vi "PH_AxisGUI_BaseClass.Find Axes of Controllers.vi"(0 "Own Motion Instance (N/A)":string="N/A", 1 "GUI Instance (N/A)":string="N/A", 2 "PH_AxisGUI_6P":bool=TRUE, 3 "PH_Sixpack_Switch":bool=TRUE, 4 "PH_Waveplate-GUI_6P":bool=TRUE, 5 "error in":errorcluster, 7 "PH_4_Pos_Selector":bool=TRUE, 9 "PH_Revolver-GUI_6P":bool=TRUE) -> (17 "Result":T2(array[cluster]), 19 "error out":errorcluster)   [LabVIEW 2014, in "PH_AxisGUI_BaseClass.lvlib"]
doc: "This VI reads out the database: It searches for all Motion and related GUI instances. \n\nIf \"GUI Instance (N/A)\" is connected, THIS GUI instance is kicked out of the Results.\n\nIf \"Own 6P Controller Instance (N/A)\" is connected, only GUIs of this THIS instances are given out; otherwise all.\n\nThe results are a multi-line three column olutput: \n1. columns is the motion instance,\n2. column is the axis GUI name, \n3. column is the motor number."
uses:
  PH_AxisGUI_BaseClass.lvlib
  PH_Stepmotor_BaseClass/PH_Stepmotor_BaseClass.Axis Address.ctl
  PH_Common/PH_Common.lvlib
  PH_Stepmotor_BaseClass/PH_Stepmotor_BaseClass.lvlib
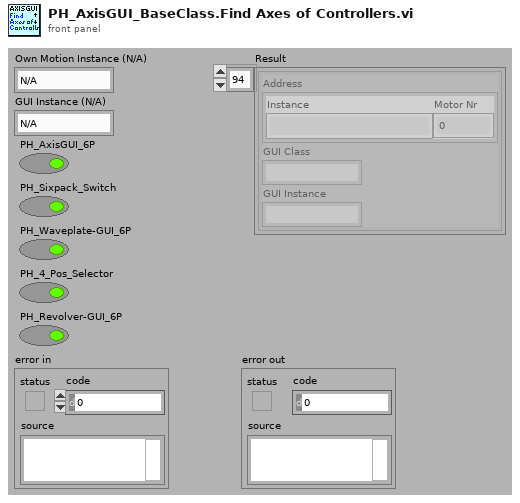
[diagram p1: front panel]
types:
  T1 = typedef "PH_Stepmotor_BaseClass.lvlib/PH_Stepmotor_BaseClass.Axis Address.ctl" = cluster{"Instance":string, "Motor Nr":i32}
  T2 = cluster{"Address":T1, "GUI Class":string, "GUI Instance":string}[]
  T3 = cluster{"Address":T1, "GUI Class":string, "GUI Instance":string}
  T4 = typedef "PH_AxisGUI_BaseClass.lvlib/PH_AxisGUI_BaseClass.Database Entry.ctl" = cluster{"Address":T1, "Name":string, "Label \"Back\"":string, "Labell \"Forth\"":string}
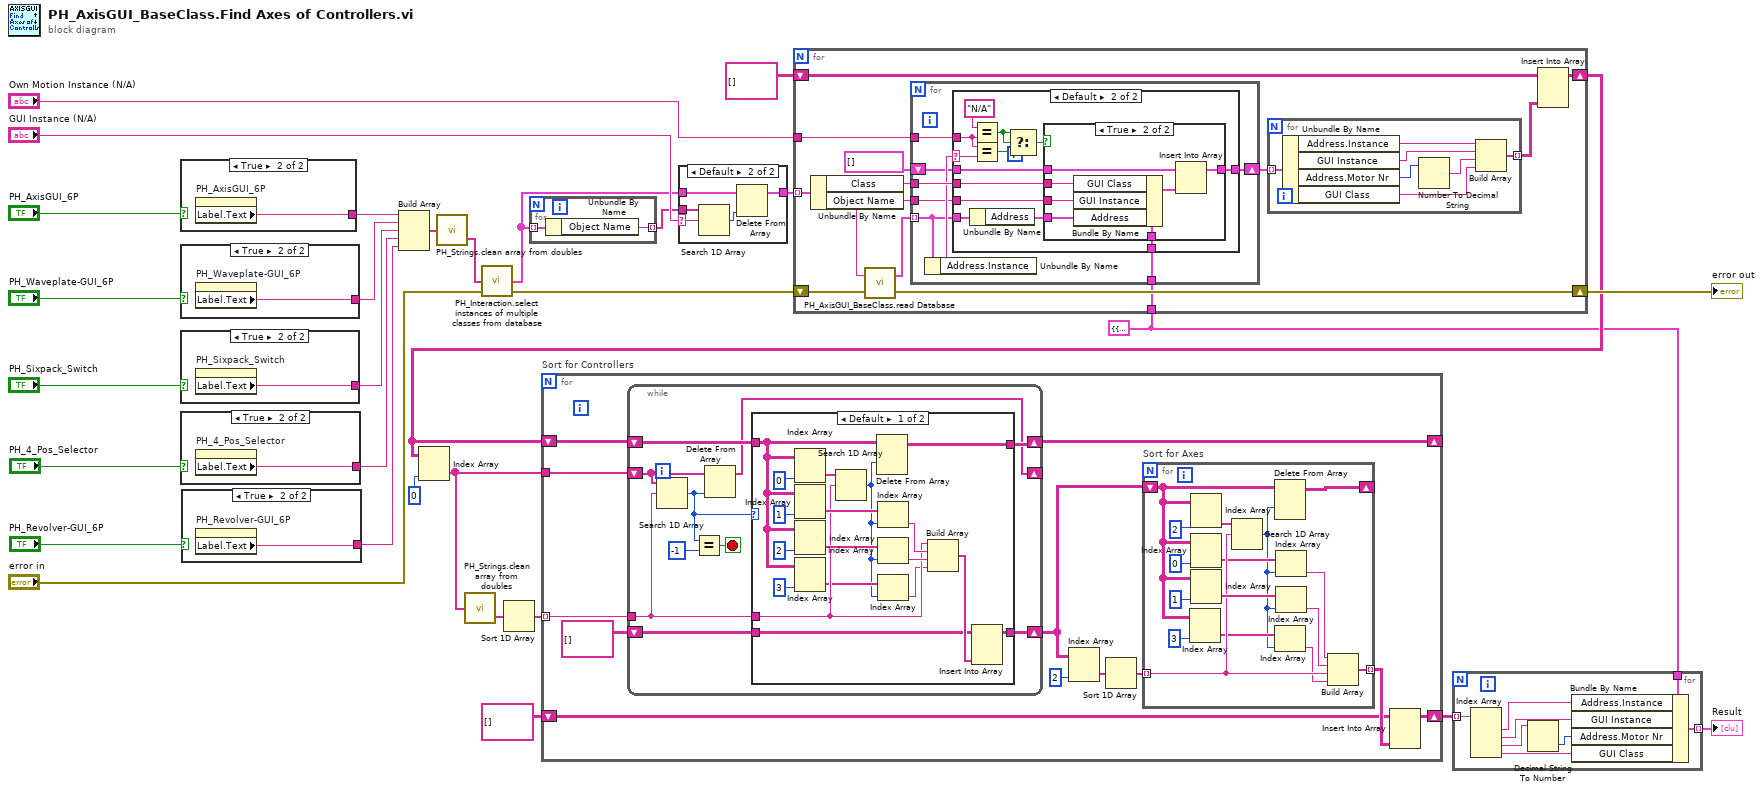
[diagram p0: block diagram]
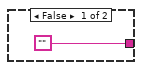
[diagram p3: hidden frame]
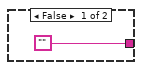
[diagram p4: hidden frame]
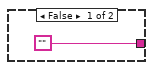
[diagram p5: hidden frame]
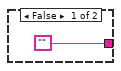
[diagram p6: hidden frame]
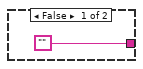
[diagram p7: hidden frame]
diagram:
  w3 = T3 {"Address"={"Instance"="N/A", "Motor Nr"=0}, "GUI Class"="", "GUI Instance"=""}
  n1 = case shown="True" "PH_AxisGUI_6P" {
    tunnel: ["" w32] -> w16
    frame False {
    }
    frame True {
      n2 = property on="PH_AxisGUI_6P" class="Bool (strict)"() -> ("Label.Text"=w32:string)  [unwired: 2 in, 2 out]
    }
  }
  n3 = case shown="True" "PH_Waveplate-GUI_6P" {
    tunnel: ["" w34] -> w20
    frame False {
    }
    frame True {
      n4 = property on="PH_Waveplate-GUI_6P" class="Bool (strict)"() -> ("Label.Text"=w34:string)  [unwired: 2 in, 2 out]
    }
  }
  n5 = case shown="True" "PH_Sixpack_Switch" {
    tunnel: ["" w36] -> w17
    frame False {
    }
    frame True {
      n6 = property on="PH_Sixpack_Switch" class="Bool (strict)"() -> ("Label.Text"=w36:string)  [unwired: 2 in, 2 out]
    }
  }
  n7 = case shown="True" "PH_4_Pos_Selector" {
    tunnel: ["" w38] -> w14
    frame False {
    }
    frame True {
      n8 = property on="PH_4_Pos_Selector" class="Bool (strict)"() -> ("Label.Text"=w38:string)  [unwired: 2 in, 2 out]
    }
  }
  n9 = case shown="True" "PH_Revolver-GUI_6P" {
    tunnel: ["" w40] -> w12
    frame False {
    }
    frame True {
      n10 = property on="PH_Revolver-GUI_6P" class="Bool (strict)"() -> ("Label.Text"=w40:string)  [unwired: 2 in, 2 out]
    }
  }
  n11 = Build Array(w16, w20, w17, w14, w12) -> (w19:string[])
  n12 = call "PH_Strings.clean array from doubles.vi"("Array Input"=w19) -> ("Cleaned Array Output"=w18:string[])  [unwired: 1 out]
  n13 = call "PH_Interaction.select instances of multiple classes from database.vi"("error in (no error)"="error in", "Classes Input"=w18) -> ("error out"=w28:errorcluster, "Query Result"=w9:cluster{"Object Name":string, "Class":string}[])  [unwired: 2 in]
  n14 = for {
    tunnel: w9 -> [w42] mode=indexing
    tunnel: [w41] -> w8 mode=indexing
    n15 = Unbundle By Name(w42) -> ("Object Name"=w41:string)
  }
  n16 = case shown="Default" "GUI Instance (N/A)" {
    selector: "GUI Instance (N/A)" -> [_ w46]
    tunnel: w9 -> [w43 w45]
    tunnel: [w43 w48] -> w7
    tunnel: w8 -> [_ w44]
    frame "", "N/A" {
    }
    frame Default {
      n17 = Search 1D Array(1D array=w44, element=w46) -> (index of element=w47:i32)  [unwired: 1 in]
      n18 = Delete From Array(array=w45, index=w47) -> (array with subset deleted=w48:cluster{"Object Name":string, "Class":string}[])  [unwired: 1 in, 1 out]
    }
  }
  n19 = for {
    shift-right: [w56] -> w29
    shift-left: w28 -> [w57]
    tunnel: "Own Motion Instance (N/A)" -> [w61]
    tunnel: w7 -> [w60] mode=indexing
    tunnel: w3 -> [w55]
    shift-right: [w51] -> w5
    shift-left: string[][] [] ("Array") -> [w50]
    n20 = Unbundle By Name(w60) -> ("Class"=w58:string, "Object Name"=w49:string)
    n21 = call "PH_AxisGUI_BaseClass.read Database.vi"("error in (no error)"=w57, "DB Entry to read"=w49) -> ("error out"=w56:errorcluster, "DB EntriesArray"=w59:T4[])
    n22 = for {
      tunnel: w59 -> [w71] mode=indexing
      tunnel: w58 -> [w76]
      shift-right: [w74] -> w53
      shift-left: T2 [] -> [w73]
      tunnel: w61 -> [w72]
      tunnel: w55 -> [w70]
      tunnel: w49 -> [w69]
      n23 = Unbundle By Name(w71) -> ("Address.Instance"=w75:string)
      n24 = case shown="Default" w75 {
        selector: w75 -> [_ w83]
        tunnel: w76 -> [_ w90]
        tunnel: [w77 w89] -> w74
        tunnel: w73 -> [w77 w88]
        tunnel: w72 -> [_ w84]
        tunnel: w71 -> [_ w80]
        tunnel: w70 -> [_ w79]
        tunnel: w69 -> [_ w78]
        frame "", "N/A" {
        }
        frame Default {
          n25 = Unbundle By Name(w80) -> ("Address"=w81:T1)
          n26 = Equal?(x="N/A" ("y"), y=w84) -> (x = y?=w86:bool)
          n27 = Equal?(x=w84, y=w83) -> (x = y?=w82:bool)
          n28 = Select(t=w86, s=w86, f=w82) -> (s? t:f=w85:bool)
          n29 = case shown="True" w85 {
            tunnel: w90 -> [_ w96]
            tunnel: [w91 w98] -> w89
            tunnel: w88 -> [w91 w97]
            tunnel: w81 -> [_ w95]
            tunnel: w79 -> [_ w93]
            tunnel: w78 -> [_ w92]
            frame False {
            }
            frame True {
              n30 = Bundle By Name(cluster=w93, "GUI Class"=w96, "GUI Instance"=w92, "Address"=w95) -> (w94:T3)
              n31 = Insert Into Array(array=w97, new element=w94) -> (w98:T2)  [unwired: 1 in]
            }
          }
        }
      }
    }
    n32 = for {
      tunnel: w53 -> [w68] mode=indexing
      tunnel: [w64] -> w52 mode=indexing
      n33 = Unbundle By Name(w68) -> ("Address.Instance"=w66:string, "GUI Instance"=w62:string, "Address.Motor Nr"=w67:i32, "GUI Class"=w63:string)
      n34 = Number To Decimal String(number=w67) -> (decimal integer string=w65:string)  [unwired: 1 in]
      n35 = Build Array(w66, w62, w65, w63) -> (w64:string[])
    }
    n36 = Insert Into Array(array=w50, new element=w52) -> (w51:string[][])  [unwired: 2 in]
  }
  "error out" <- w29
  n37 = Index Array(array=w5, index (col)=0 ("disabled index (col)")) -> (element=w24:string[])  [unwired: 1 in]
  n38 = call "PH_Strings.clean array from doubles.vi"("Array Input"=w24) -> ("Cleaned Array Output"=w26:string[])  [unwired: 1 out]
  n39 = Sort 1D Array(array=w26) -> (sorted array=w25:string[])
  n40 = for "Sort for Controllers" {
    tunnel: w25 -> [w110] mode=indexing
    shift-right: [w107] -> _
    shift-left: w5 -> [w108]
    tunnel: w24 -> [w109]
    shift-right: [w102] -> w2
    shift-left: string[][] [] ("Array") -> [w100]
    n41 = while {
      shift-right: [w130] -> _
      shift-left: w109 -> [w136]
      tunnel: w110 -> [w131]
      shift-right: [w132] -> w107
      shift-left: w108 -> [w133]
      shift-right: [w129] -> w103
      shift-left: string[][] [] ("Array") -> [w128]
      stop <- w134 stop-if-true
      n42 = Search 1D Array(1D array=w136, element=w131) -> (index of element=w127:i32)  [unwired: 1 in]
      n43 = Equal?(x=w127, y=-1) -> (x = y?=w134:bool)
      n44 = Delete From Array(array=w136, index=w127) -> (array with subset deleted=w130:string[])  [unwired: 1 in, 1 out]
      n45 = case shown="Default" w127 {
        tunnel: w133 -> [w139 w155]
        tunnel: [w146 w155] -> w132
        tunnel: w131 -> [w145 _]
        tunnel: [w143 w156] -> w129
        tunnel: w128 -> [w142 w156]
        frame Default {
          n46 = Index Array(array=w139, index (col)=0 ("disabled index (col)")) -> (element=w153:string[])  [unwired: 1 in]
          n47 = Index Array(array=w139, index (col)=1 ("disabled index (col)")) -> (element=w149:string[])  [unwired: 1 in]
          n48 = Index Array(array=w139, index (col)=2 ("disabled index (col)")) -> (element=w151:string[])  [unwired: 1 in]
          n49 = Index Array(array=w139, index (col)=3 ("disabled index (col)")) -> (element=w140:string[])  [unwired: 1 in]
          n50 = Search 1D Array(1D array=w153, element=w145) -> (index of element=w138:i32)  [unwired: 1 in]
          n51 = Delete From Array(array=w139, index (row)=w138) -> (array with subset deleted=w146:string[][])  [unwired: 2 in, 1 out]
          n52 = Index Array(array=w149, index=w138) -> (element=w148:string)
          n53 = Index Array(array=w151, index=w138) -> (element=w147:string)
          n54 = Index Array(array=w140, index=w138) -> (element=w137:string)
          n55 = Build Array(w145, w148, w147, w137) -> (w144:string[])
          n56 = Insert Into Array(array=w142, new element=w144) -> (w143:string[][])  [unwired: 2 in]
        }
        frame -1 {
        }
      }
    }
    n57 = Index Array(array=w103, index (col)=2 ("disabled index (col)")) -> (element=w105:string[])  [unwired: 1 in]
    n58 = Sort 1D Array(array=w105) -> (sorted array=w104:string[])
    n59 = for "Sort for Axes" {
      tunnel: w104 -> [w119] mode=indexing
      shift-right: [w123] -> _
      shift-left: w103 -> [w114]
      tunnel: [w122] -> w101 mode=indexing
      n60 = Index Array(array=w114, index (col)=3 ("disabled index (col)")) -> (element=w113:string[])  [unwired: 1 in]
      n61 = Index Array(array=w114, index (col)=2 ("disabled index (col)")) -> (element=w125:string[])  [unwired: 1 in]
      n62 = Index Array(array=w114, index (col)=0 ("disabled index (col)")) -> (element=w117:string[])  [unwired: 1 in]
      n63 = Index Array(array=w114, index (col)=1 ("disabled index (col)")) -> (element=w121:string[])  [unwired: 1 in]
      n64 = Search 1D Array(1D array=w125, element=w119) -> (index of element=w112:i32)  [unwired: 1 in]
      n65 = Delete From Array(array=w114, index (row)=w112) -> (array with subset deleted=w123:string[][])  [unwired: 2 in, 1 out]
      n66 = Index Array(array=w113, index=w112) -> (element=w111:string)
      n67 = Index Array(array=w117, index=w112) -> (element=w116:string)
      n68 = Index Array(array=w121, index=w112) -> (element=w120:string)
      n69 = Build Array(w116, w120, w119, w111) -> (w122:string[])
    }
    n70 = Insert Into Array(array=w100, new element=w101) -> (w102:string[][])  [unwired: 2 in]
  }
  n71 = for {
    tunnel: w3 -> [w164]
    tunnel: w2 -> [w163] mode=indexing
    tunnel: [w157] -> w1 mode=indexing
    n72 = Index Array(array=w163) -> (element #1=w161:string, element #2=w160:string, element #3=w158:string, element #4=w162:string)  [unwired: 4 in]
    n73 = Decimal String To Number(string=w158) -> (number=w159:i32)  [unwired: 2 in, 1 out]
    n74 = Bundle By Name(cluster=w164, "Address.Instance"=w161, "GUI Instance"=w160, "Address.Motor Nr"=w159, "GUI Class"=w162) -> (w157:T3)
  }
  "Result" <- w1
